vi "labjack.vi"(8 "error out":errorcluster, 9 "PwmDtc":dbl, 10 "Boolean":bool, 11 "Handle Out":i32) -> (0 "error out 2":errorcluster, 2 "Boolean 2":bool, 3 "Handle Out 2":i32)   [LabVIEW 2017]
panel:
  out "ErrorAddress":i32
  out "ErrorAddress 2":i32
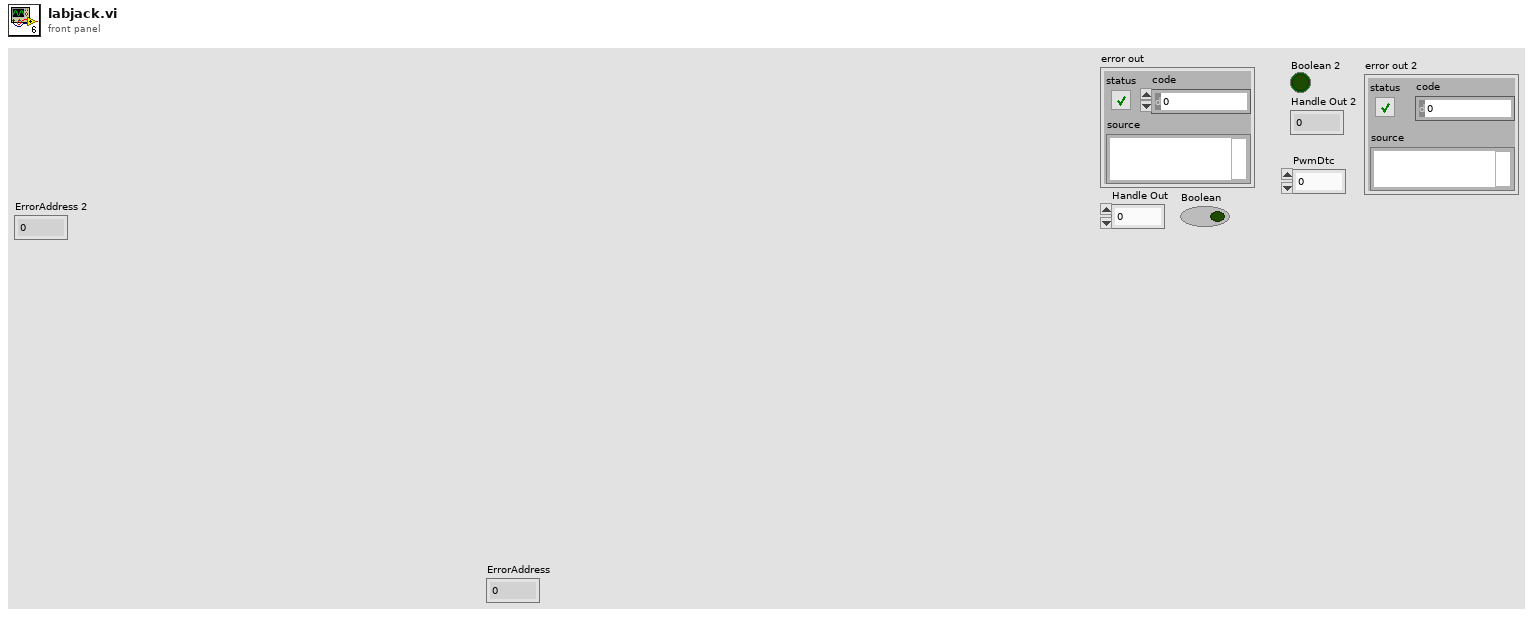
[diagram p1: front panel]
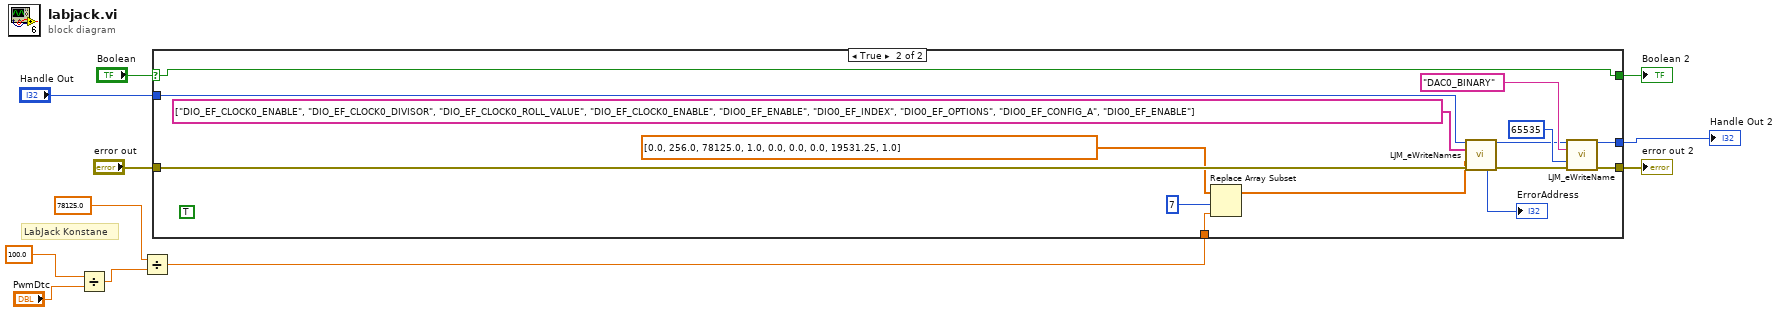
[diagram p0: block diagram]
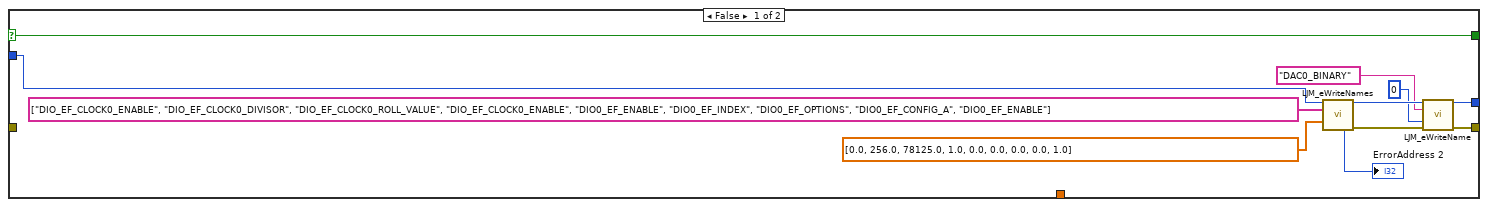
[diagram p2: hidden frame]
diagram:
  # "LabJack Konstane"
  n1 = Divide(x=100.0, y="PwmDtc") -> (x/y=w3:dbl)
  n2 = Divide(x=78125.0 ("new element/subarray"), y=w3) -> (x/y=w4:dbl)
  n3 = case shown="True" "Boolean" {
    selector: "Boolean" -> [w20 w33]
    tunnel: [w16 w29] -> w7
    tunnel: [w14 w27] -> w6
    tunnel: "Handle Out" -> [w18 w35]
    tunnel: "error out" -> [_ w34]
    tunnel: [w20 w33] -> w8
    tunnel: w4 -> [_ w23]
    frame False {
      n4 = call "LJM_eWriteNames.vi"("Handle In"=w18, "aNames"=string[] ["DIO_EF_CLOCK0_ENABLE", "DIO_EF_CLOCK0_DIVISOR", "DIO_EF_CLOCK0_ROLL_VALUE", "DIO_EF_CLOCK0_ENABLE", "DIO0_EF_ENABLE", "DIO0_EF_INDEX", "DIO0_EF_OPTIONS", "DIO0_EF_CONFIG_A", "DIO0_EF_ENABLE"], "aValuesIn"=dbl[] [0.0, 256.0, 78125.0, 1.0, 0.0, 0.0, 0.0, 0.0, 1.0]) -> ("Handle Out"=w17:i32, "ErrorAddress"=→"ErrorAddress 2":i32, "error out"=w15:errorcluster)  [unwired: 10 in]
      n5 = call "LJM_eWriteName.vi"("Handle In"=w17, "Name"="DAC0_BINARY", "Value"=u32 0, "error in"=w15) -> ("Handle Out"=w16:i32, "error out"=w14:errorcluster)  [unwired: 10 in]
    }
    frame True {
      (unwired) TRUE
      n6 = Replace Array Subset(array=dbl[] [0.0, 256.0, 78125.0, 1.0, 0.0, 0.0, 0.0, 19531.25, 1.0] ("aValuesIn"), new element=w23, index=7) -> (w25:dbl[])
      n7 = call "LJM_eWriteNames.vi"("Handle In"=w35, "aNames"=string[] ["DIO_EF_CLOCK0_ENABLE", "DIO_EF_CLOCK0_DIVISOR", "DIO_EF_CLOCK0_ROLL_VALUE", "DIO_EF_CLOCK0_ENABLE", "DIO0_EF_ENABLE", "DIO0_EF_INDEX", "DIO0_EF_OPTIONS", "DIO0_EF_CONFIG_A", "DIO0_EF_ENABLE"], "aValuesIn"=w25, "error in"=w34) -> ("Handle Out"=w30:i32, "ErrorAddress"=→"ErrorAddress":i32, "error out"=w28:errorcluster)  [unwired: 9 in]
      n8 = call "LJM_eWriteName.vi"("Handle In"=w30, "Name"="DAC0_BINARY", "Value"=u32 65535, "error in"=w28) -> ("Handle Out"=w29:i32, "error out"=w27:errorcluster)  [unwired: 10 in]
    }
  }
  "Boolean 2" <- w8
  "Handle Out 2" <- w7
  "error out 2" <- w6
